vi "send_fixed_step_command.vi"(2 "Brake":bool, 3 "Drive mode":bool, 4 "error in":errorcluster, 5 "Right amount":dbl, 6 "Forward amount":dbl, 7 "Message":string="{\"time_step\": 1.0}") -> (0 "error out":errorcluster)   [LabVIEW 2019]
doc: "Sends a command to the Simx Simulator to control the movement of ego vehicle. Commands sent are: \n - ClosedLoopStepCommand_ID\n - SampleSensorsCommand_ID\n - EgoControl_ID"
uses:
  tools/simx_common.vi
panel:
  out "success":bool
  out "TCP Network Connection out":refnum<k5>
  out "vehicle command response":string
  # "Overview: Sends a command to the monoDrive Simulator to control the movement of ego vehicle.\n Parameters:\n  -- forward_amount: a value between -1.0 and 1.0 that determines the amount of throttle to apply\n  -- right_amount: a value between -1.0 and 1.0 that determines the steering position (-1 is left, +1 is right)\nInstructions:\nThe command used to control the throttle (forward_amount) and steering (right_amount) is used to move the ego vehicle inside the simulation. The response from the simulator will appear in the vehicle command response field below."
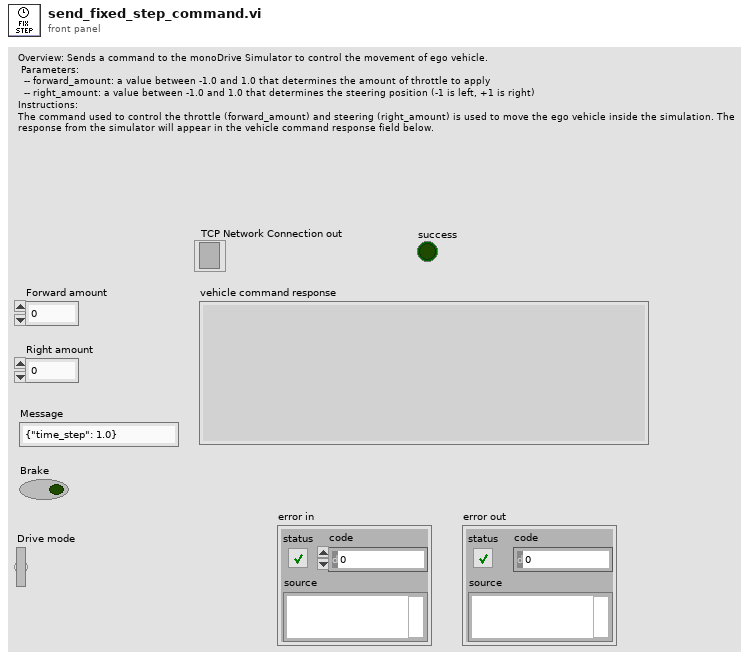
[diagram p1: front panel]
types:
  T1 = typedef "simx_connection.ctl" = cluster{"Config":T2, "Connections":T5, "Map":cluster{"lanes":cluster{"x":dbl[], "y":dbl[], "z":dbl[]}, "StartPosition":cluster{"start_points":T6, "StartRotation":dbl[], "StartLocation":dbl[]}, "Draw Map Size":T7, "DrawArea":cluster{"min_Y":dbl, "min_X":dbl, "Scale X":dbl, "Scale Y":dbl}, "Map":picture, "Map Geojson":string}}
  T2 = typedef "config.ctl" = cluster{"Trajectory":T3, "Weather":T4}
  T3 = typedef "trajectory.ctl" = cluster{"Number of frames":i32, "Frame number":i32, "Trajectory":string}
  T4 = typedef "weather.ctl" = cluster{"id":string}
  T5 = typedef "connections.ctl" = cluster{"Simulator Connection":refnum<k5>, "server_ip":string, "Port":i32, "Sensor connections":refnum<k5>[]}
  T6 = typedef "start_points.ctl" = cluster{"locations":dbl[][], "rotations":dbl[][], "type":string[]}
  T7 = typedef "LVBoundsTypeDef.ctl" = cluster{"Width":u32, "Height":u32}
  T8 = cluster{"forward_amount":dbl, "right_amount":dbl, "brake_amount":i16, "drive_mode":i16}
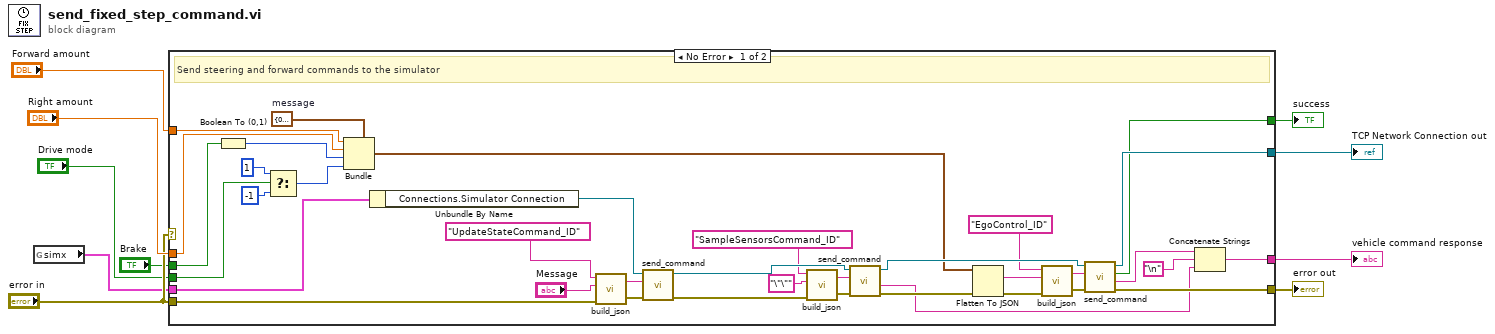
[diagram p0: block diagram]
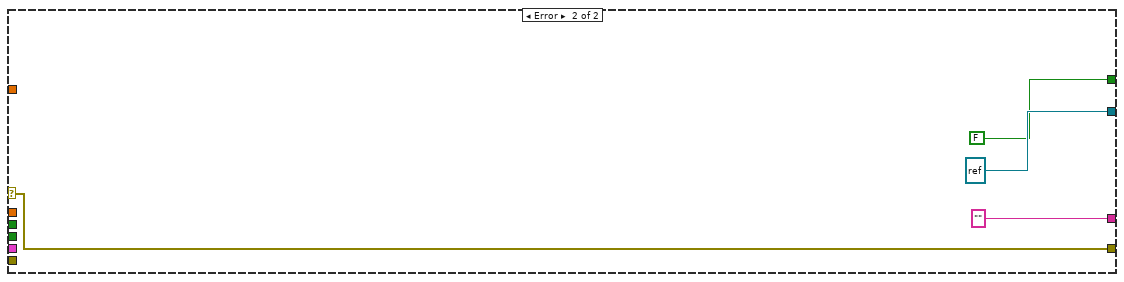
[diagram p2: hidden frame]
diagram:
  n1 = global read "simx_common.vi" "simx"() -> (w1:T1)
  n2 = case shown="No Error" "error in" {
    selector: "error in" -> [_ w51]
    tunnel: [w30 w51] -> w10
    tunnel: "Right amount" -> [w47 _]
    tunnel: "Forward amount" -> [w46 _]
    tunnel: [w39 "" ("response")] -> w7
    tunnel: [w22 refnum<k5> refnum ("TCP Network Connection Out")] -> w6
    tunnel: [w11 FALSE ("success")] -> w5
    tunnel: "error in" -> [w37 _]
    tunnel: "Brake" -> [w45 _]
    tunnel: "Drive mode" -> [w44 _]
    tunnel: w1 -> [w32 _]
    frame No Error {
      w15 = T8 {"forward_amount"=0.0, "right_amount"=0.0, "brake_amount"=0, "drive_mode"=0}  # message
      # "Send steering and forward commands to the simulator"
      n3 = Boolean To (0,1)(Boolean=w45) -> (0, 1=w19:i16)
      n4 = Select(t=1, s=w44, f=-1) -> (s? t:f=w16:i32)
      n5 = Bundle(cluster=w15, "forward_amount"=w46, "right_amount"=w47, "brake_amount"=w19, "drive_mode"=w16) -> (w14:T8)
      n6 = Unbundle By Name(w32) -> ("Connections.Simulator Connection"=w31:refnum<k5>)
      n7 = call "build_json.vi"("error in"=w37, "Message"="Message", "Command_ID"="UpdateStateCommand_ID") -> ("error out"=w34:errorcluster, "JSON Out"=w33:string)  [unwired: 1 in]
      n8 = call "send_command.vi"("error in"=w34, "JSON Command"=w33, "TCP Network Connection in"=w31) -> ("error out"=w27:errorcluster, "TCP Network Connection Out"=w26:refnum<k5>)  [unwired: 1 in, 2 out]
      n9 = call "build_json.vi"("error in"=w27, "Message"="\"\"" ("message"), "Command_ID"="SampleSensorsCommand_ID" ("type")) -> ("error out"=w29:errorcluster, "JSON Out"=w28:string)  [unwired: 1 in]
      n10 = call "send_command.vi"("error in"=w29, "JSON Command"=w28, "TCP Network Connection in"=w26) -> ("error out"=w24:errorcluster, "Response"=w23:string, "TCP Network Connection Out"=w25:refnum<k5>)  [unwired: 1 in, 1 out]
      n11 = Flatten To JSON(anything=w14, error in (no error)=w24) -> (JSON string=w12:string, 11:w35:errorcluster)  [unwired: 1 in]
      n12 = call "build_json.vi"("error in"=w35, "Message"=w12, "Command_ID"="EgoControl_ID") -> ("error out"=w43:errorcluster, "JSON Out"=w42:string)  [unwired: 1 in]
      n13 = call "send_command.vi"("error in"=w43, "JSON Command"=w42, "TCP Network Connection in"=w25) -> ("error out"=w30:errorcluster, "Response"=w41:string, "Success"=w11:bool, "TCP Network Connection Out"=w22:refnum<k5>)  [unwired: 1 in]
      n14 = Concatenate Strings(w41, "\n", w23) -> (w39:string)
    }
    frame Error {
    }
  }
  "vehicle command response" <- w7
  "TCP Network Connection out" <- w6
  "error out" <- w10
  "success" <- w5
